vi "ParseVectorFile.TestLauncher.vi"() -> ()   [LabVIEW 2019, in "ParseVectorFile.lvclass"]
uses:
  ParseVectorFile.lvclass
  <vilib>/JKI/JKI SMO/SMO/Typedefs/SMOState --Enum.ctl
  Typedefs/PublicEvents--ParseVectorFile.ParsedData.ctl
  Image/SVGImage.lvclass
  C:/Program Files (x86)/National Instruments/LabVIEW 2019/vi.lib/JKI/JKI SMO/SMO/SMO.lvclass
  <vilib>/JKI/JKI SMO/SMO/SMO.lvclass/SMO.ctl
  Image/SVGImage.lvclass/SVGImage.ctl
  <vilib>/JKI/JKI SMO/SMO/Private/ReftoDVR--SMO.vi
  <vilib>/JKI/JKI SMO/SMO/SMO.lvclass
  ParsePaths/Path.lvclass
  Rectangle/Rectangle.lvclass
  Dot/Dot.lvclass
panel:
  out "ParsedData":T1
  in  "SVG Path Synch":path
  in  "SVG Path":path
  out "Height":dbl
  out "Rects":i32
  out "Paths":i32
  out "SMO State":T2
  out "error out":errorcluster
  in  "Stop":bool
  # "Parse Vector File Test Launcher"
  # "For instructions on how to use the JKI State Machine Objects, examples and video tutorials, visit:\nhttp://jki.net/state-machine-objects/\n\nJKI State Machine Objects™\nhttp://jki.net/state-machine-objects/\nCopyright (C) 2005-2015, JKI <info@jki.net>\nALL RIGHTS RESERVED"
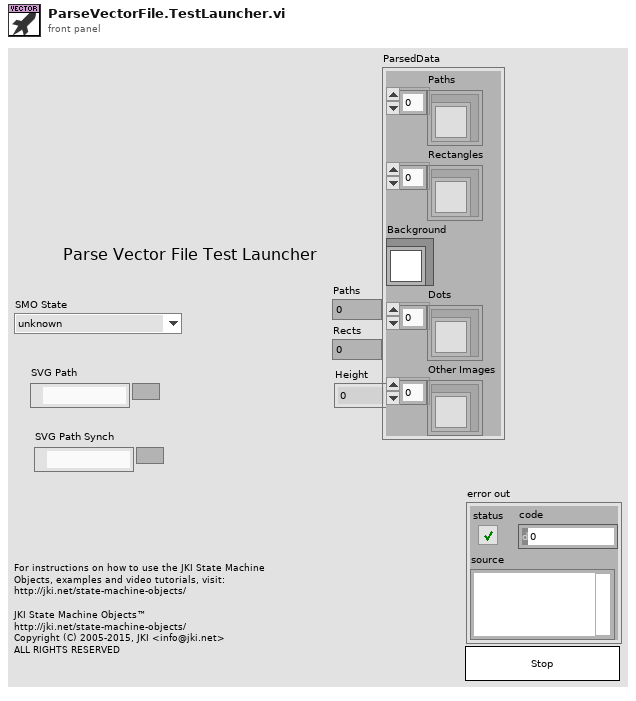
[diagram p1: front panel]
types:
  T1 = typedef "ParseVectorFile.lvclass/PublicEvents--ParseVectorFile.ParsedData.ctl" = cluster{"Paths":refnum<class "Path.lvclass">[], "Rectangles":refnum<class "Rectangle.lvclass">[], "Background":refnum<class "SVGImage.lvclass">, "Dots":refnum<class "Dot.lvclass">[], "Other Images":refnum<class "SVGImage.lvclass">[]}
  T2 = typedef "SMO.lvclass/SMOState --Enum.ctl" = enum16{"unknown", "Created", "Started", "Stopped"}
  T3 = typedef "SMO.lvclass/Public Events.ctl" = cluster{"Error":refnum<user-event>, "State":refnum<user-event>, "Reserve State":refnum<user-event>}
  T4 = typedef "ParseVectorFile.lvclass/PublicEvents--Cluster.ctl" = cluster{"ParsedData":refnum<user-event>}
  T5 = cluster{"Event Registration Refnum":refnum<event-registration>}
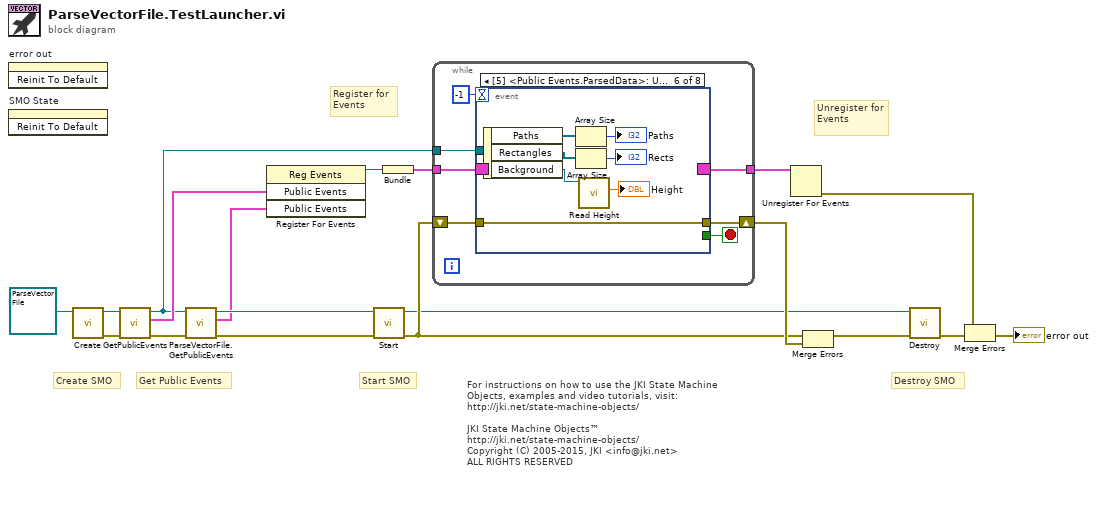
[diagram p0: block diagram]
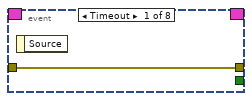
[diagram p2: hidden frame]
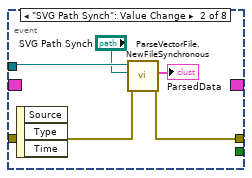
[diagram p3: hidden frame]
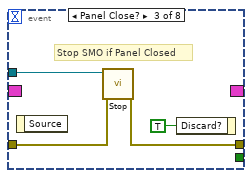
[diagram p4: hidden frame]
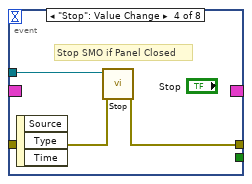
[diagram p5: hidden frame]
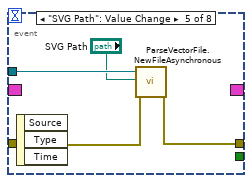
[diagram p6: hidden frame]
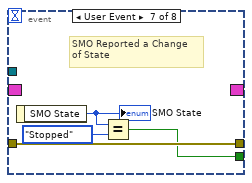
[diagram p7: hidden frame]
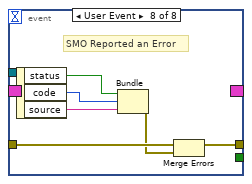
[diagram p8: hidden frame]
diagram:
  # "For instructions on how to use the JKI State Machine Objects, examples and video tutorials, visit:\nhttp://jki.net/state-machine-objects/\n\nJKI State Machine Objects™\nhttp://jki.net/state-machine-objects/\nCopyright (C) 2005-2015, JKI <info@jki.net>\nALL RIGHTS RESERVED"
  # "Get Public Events"
  # "Start SMO"
  # "Destroy SMO"
  # "Create SMO"
  # "Unregister for Events"
  # "Register for Events"
  n1 = invoke on="error out" class="Clust (strict)" method="Reinit To Default"() -> ()  [unwired: 3 in, 3 out]
  n2 = invoke on="SMO State" class="Enum (strict)" method="Reinit To Default"() -> ()  [unwired: 3 in, 3 out]
  n3 = call <vilib>:"Create.vi"("SMO"=refnum<class "ParseVectorFile.lvclass"> refnum ("SMO.Template.lvclass")) -> ("error out"=w8:errorcluster, "SMO out"=w9:refnum<class "ParseVectorFile.lvclass">)  [unwired: 8 in, 1 out]
  n4 = call <vilib>:"GetPublicEvents.vi"("error in (no error)"=w8, "SMO"=w9) -> ("error out"=w5:errorcluster, "Public Events"=w7:T3, "SMO out"=w3:refnum<class "ParseVectorFile.lvclass">)  [unwired: 7 in]
  n5 = call "ParseVectorFile.GetPublicEvents.vi"("error in (no error)"=w5, "ParseVectorFile"=w3) -> ("error out"=w4:errorcluster, "Public Events"=w1:T4, "ParseVectorFile out"=w2:refnum<class "ParseVectorFile.lvclass">)  [unwired: 7 in]
  n6 = register-events(w7, w1) -> (reference out=w6:refnum<event-registration>)  [unwired: 2 in, 1 out]
  n7 = call <vilib>:"Start.vi"("error in (no error)"=w4, "SMO"=w2) -> ("error out"=w12:errorcluster, "SMO out"=w10:refnum<class "ParseVectorFile.lvclass">)  [unwired: 8 in]
  n8 = Bundle("Event Registration Refnum"=w6) -> (w18:T5)  [unwired: 1 in]
  n9 = while {
    shift-right: [w25] -> w17
    shift-left: w12 -> [w24]
    tunnel: w18 -> [w23]
    tunnel: [w22] -> w19
    tunnel: w3 -> [w21]
    stop <- w26 stop-if-true
    n10 = event shown="[5] <Public Events.ParsedData>: User Event" {
      selector: w23 -> [_ _ _ _ _ _ _ _]
      dyn-events: [_ _ _ _ _ _ _ _] -> w22
      timeout: -1 -> [_ _ _ _ _ _ _ _]
      tunnel: [_ _ _ _ _ _ w51 _] -> w26
      tunnel: w21 -> [_ w32 w36 w39 w43 _ _ _]
      tunnel: [w27 w31 w35 w38 w40 w44 w54 w58] -> w25
      tunnel: w24 -> [w27 w30 w34 w37 w41 w44 w54 w56]
      event Timeout {
        n11 = event-data() -> ()  [unwired: 1 in, 1 out]
      }
      event "SVG Path Synch": Value Change {
        n12 = event-data() -> ()  [unwired: 1 in, 3 out]
        n13 = call "ParseVectorFile.NewFileSynchronous.vi"("error in (no error)"=w30, "Path"="SVG Path Synch", "ParseVectorFile"=w32) -> ("error out"=w31:errorcluster, "ParsedData"=→"ParsedData":T1)  [unwired: 6 in, 1 out]
      }
      event Panel Close? {
        # "Stop SMO if Panel Closed"
        n14 = event-data() -> ()  [unwired: 1 in, 1 out]
        n15 = call <vilib>:"Stop.vi"("error in (no error)"=w34, "SMO"=w36) -> ("error out"=w35:errorcluster)  [unwired: 8 in, 1 out]
        n16 = event-data("Discard?"=TRUE ("OK")) -> ()  [unwired: 1 in, 1 out]
      }
      event "Stop": Value Change {
        # "Stop SMO if Panel Closed"
        n17 = event-data() -> ()  [unwired: 1 in, 3 out]
        n18 = call <vilib>:"Stop.vi"("error in (no error)"=w37, "SMO"=w39) -> ("error out"=w38:errorcluster)  [unwired: 8 in, 1 out]
      }
      event "SVG Path": Value Change {
        n19 = event-data() -> ()  [unwired: 1 in, 3 out]
        n20 = call "ParseVectorFile.NewFileAsynchronous.vi"("error in (no error)"=w41, "NewFile"="SVG Path", "ParseVectorFile"=w43) -> ("error out"=w40:errorcluster)  [unwired: 7 in, 1 out]
      }
      event User Event {
        n21 = event-data() -> ("Paths"=w50:refnum<class "Path.lvclass">[], "Rectangles"=w49:refnum<class "Rectangle.lvclass">[], "Background"=w46:refnum<class "SVGImage.lvclass">)  [unwired: 1 in]
        n22 = Array Size(array=w50) -> (size(s)=→"Paths":i32)
        n23 = Array Size(array=w49) -> (size(s)=→"Rects":i32)
        n24 = call "Read Height.vi"("Image in"=w46) -> ("Height"=→"Height":dbl)  [unwired: 8 in, 2 out]
      }
      event User Event {
        # "SMO Reported a Change\nof State"
        n25 = event-data() -> ("SMO State"=w53:T2)  [unwired: 1 in]
        "SMO State" <- w53
        n26 = Equal?(x=w53, y=SMOState_--Enum."Stopped") -> (x = y?=w51:bool)
      }
      event User Event {
        # "SMO Reported an Error"
        n27 = event-data() -> ("status"=w57:bool, "code"=w60:i32, "source"=w59:string)  [unwired: 1 in]
        n28 = Bundle("status"=w57, "code"=w60, "source"=w59) -> (w55:errorcluster)  [unwired: 1 in]
        n29 = Merge Errors(w56, w55) -> (w58:errorcluster)
      }
    }
  }
  n30 = Unregister For Events(event registration refnum=w19) -> (error out=w16:errorcluster)  [unwired: 1 in]
  n31 = Merge Errors(w12, w17) -> (w11:errorcluster)
  n32 = call <vilib>:"Destroy.vi"("error in (no error)"=w11, "SMO"=w10) -> ("error out"=w14:errorcluster)  [unwired: 9 in]
  n33 = Merge Errors(w16, w14) -> (→"error out":errorcluster)
